vi "Configure Ref Clock Source.vi"(8 "error in (no error)":errorcluster, 9 "reference clock source (Internal)":i32(ring) items=["Internal"=0, "External"=1, "RTSI Clock"=101], 11 "CS++Fgen in":refnum<class "CS++Fgen.lvclass">) -> (0 "error out":errorcluster, 3 "CS++Fgen out":refnum<class "CS++Fgen.lvclass">)   [LabVIEW 2015, in "CS++Fgen.lvlib" / "CS++Fgen.lvclass"]
doc: "This VI configures the function generator's reference clock source. The function generator uses the reference clock to derive frequencies and sample rates when generating output."
uses:
  CS++Fgen.lvclass
  CSPP_Core/Classes/CS++ProcessVariables/ProcessVariable/PV.lvclass
  PV-Enum.ctl
  CSPP_Core/Classes/CS++ProcessVariables/ProcessVariable/PV.lvclass/PV.ctl
  CS++Fgen.lvclass/CS++Fgen.ctl
  CSPP_Core/Classes/CS++ProcessVariables/ProcessVariable/Write Data.vi
  CSPP_Core/Classes/CS++ProcessVariables/ProcessVariable/Write Timestamp.vi
  CSPP_Core/Classes/CS++ProcessVariables/ProcessVariable/Write Quality.vi
  CSPP_Core/Classes/CS++ProcessVariables/ProcessVariable/Write status.vi
  CSPP_Core/Classes/CS++ProcessVariables/PVConnection/PVConnection.lvclass
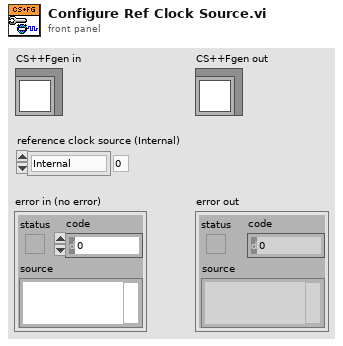
[diagram p1: front panel]
types:
  T1 = typedef "CS++Fgen.lvlib/CS++Fgen.lvclass/PV-Enum.ctl" = enum16{"AM-ModulationDepth", "AM-ModulationFrequency", "FM-ModulationFrequency", "FP-PeakDeviation", "SampleRate", "TriggerRate", "AM-ModulationWaveform", "FM-ModulationWaveform", "OutputMode", "ReferenceClockSource", "SampleClockSource", "SampleClockOutputEnabled"}
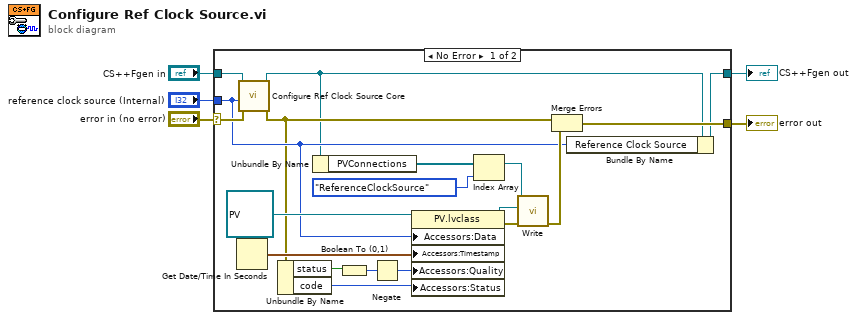
[diagram p0: block diagram]
diagram:
  n1 = case shown="No Error" "error in (no error)" {
    selector: "error in (no error)" -> [w23 w26]
    tunnel: [w10 w26] -> w4
    tunnel: [w8 w25] -> w2
    tunnel: "CS++Fgen in" -> [w24 w25]
    tunnel: "reference clock source (Internal)" -> [w12 _]
    frame No Error {
      n2 = Get Date/Time In Seconds() -> (seconds since 1Jan1904=w22:timestamp)
      n3 = call-dynamic "Configure Ref Clock Source Core.vi"("error in (no error)"=w23, "reference clock source (Internal)"=w12, "CS++Fgen in"=w24) -> ("error out"=w11:errorcluster, "CS++Fgen out"=w9:refnum<class "CS++Fgen.lvclass">)  [unwired: 7 in]
      n4 = Unbundle By Name(w11) -> ("status"=w17:bool, "code"=w15:i32)
      n5 = Unbundle By Name(w9) -> ("PVConnections"=w13:refnum<class "PVConnection.lvclass">[])
      n6 = Boolean To (0,1)(Boolean=w17) -> (0, 1=w16:i16)
      n7 = Negate(x=w16) -> (-x=w14:i16)
      n8 = property class="PV.lvclass"(reference=refnum<class "PV.lvclass"> refnum ("PV"), "Accessors:Data"=w12, "Accessors:Timestamp"=w22, "Accessors:Quality"=w14, "Accessors:Status"=w15) -> (reference out=w19:refnum<class "PV.lvclass">, error out=w20:errorcluster)  [unwired: 1 in]
      n9 = Index Array(array=w13, index=PV-Enum."ReferenceClockSource" ("PV-Enum")) -> (element=w7:refnum<class "PVConnection.lvclass">)
      n10 = call "Write.vi"("error in (no error)"=w20, "PV"=w19, "PVConnection in"=w7) -> ("error out"=w18:errorcluster)  [unwired: 7 in, 1 out]
      n11 = Merge Errors(w11, w18) -> (w10:errorcluster)
      n12 = Bundle By Name(cluster=w9, "Reference Clock Source"=w12) -> (w8:refnum<class "CS++Fgen.lvclass">)
    }
    frame Error {
    }
  }
  "error out" <- w4
  "CS++Fgen out" <- w2
